vi "U32ToBigInt.vi"(1 "U32 (<1e9)":u32) -> (0 "Big Number":cluster{"P/N":bool, "Array":dbl[]} {"Array" format="%#_16g"})   [LabVIEW 2023]
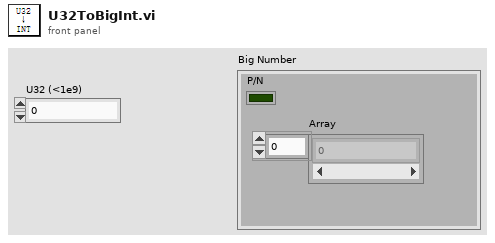
[diagram p1: front panel]
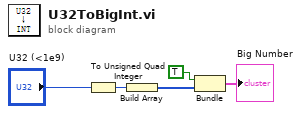
[diagram p0: block diagram]
diagram:
  n1 = To Unsigned Quad Integer(1:"U32 (<1e9)") -> (0:w2:u64)
  n2 = Build Array(w2) -> (w3:u64[])
  n3 = Bundle(TRUE, w3) -> (→"Big Number":cluster{bool, u64[]})  [unwired: 1 in]
